vi "replace AO wf param.vi"(0 "Digital Freq (Hz)":dbl, 1 "Digital DC (%)":dbl, 2 "Digital phase":dbl, 3 "Sampling frequency (Hz)":dbl, 4 "Digital time offset (s)":dbl, 5 "index of DO wave":i32, 8 "padding value":dbl) -> ()   [LabVIEW 2015]
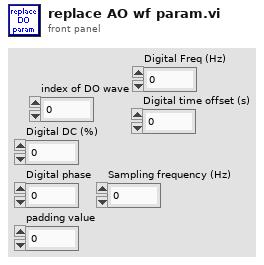
[diagram p1: front panel]
types:
  T1 = cluster{"AO parameters":cluster{"AOtab":dbl, "Repeats":dbl, "Cycles":dbl, "Start amplitude (V)":dbl, "Baseline (V)":dbl, "Step size (V)":dbl, "DC (%)":dbl, "Sampling frequency (Hz)":dbl, "Period (ms)":dbl, "Offset (V)":dbl, "Amplitude (V)":dbl, "Frequency":dbl, "Tri Repeats":dbl, "Cycle length (s)":dbl, "Pulses":dbl, "Matlab wave number":dbl, "Tri phase":dbl, "padding value":dbl}[], "DO parameters":cluster{"Digital DC (%)":dbl, "Digital phase":dbl, "Digital Freq (Hz)":dbl, "Sampling frequency (Hz)":dbl, "Digital time offset (s) ":dbl, "padding value":dbl}[]}
  T2 = cluster{"Digital DC (%)":dbl, "Digital phase":dbl, "Digital Freq (Hz)":dbl, "Sampling frequency (Hz)":dbl, "Digital time offset (s) ":dbl, "padding value":dbl}[]
  T3 = cluster{"Digital DC (%)":dbl, "Digital phase":dbl, "Digital Freq (Hz)":dbl, "Sampling frequency (Hz)":dbl, "Digital time offset (s) ":dbl, "padding value":dbl}
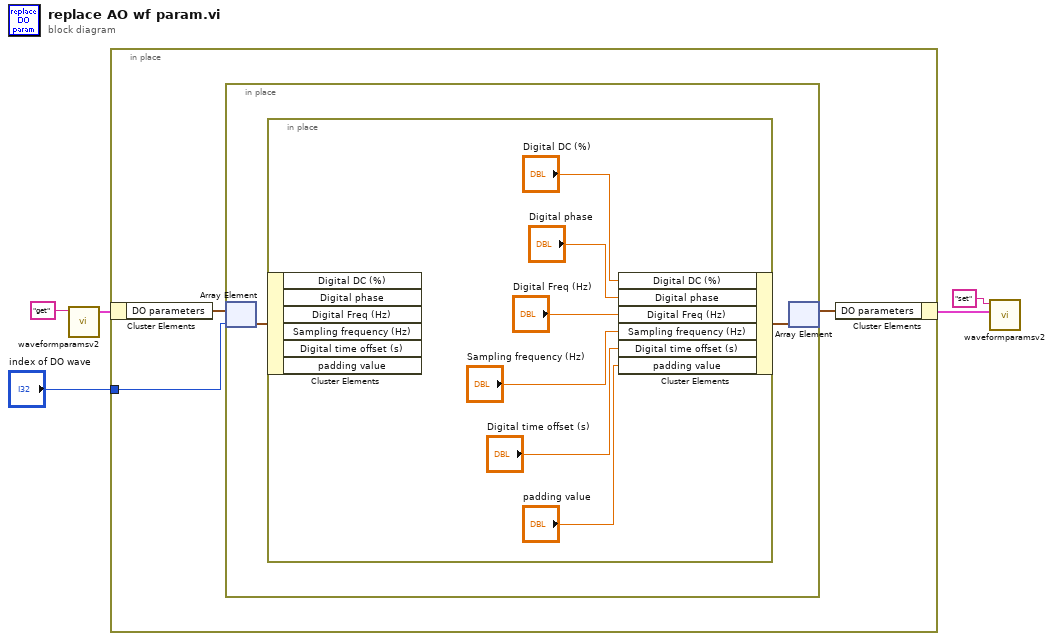
[diagram p0: block diagram]
diagram:
  n1 = call "waveformparamsv2.vi"("command"="get") -> ("Params out"=w3:T1)  [unwired: 4 in, 2 out]
  n2 = in-place {
    in-place-border: "index of DO wave" -> [w6]
    n3 = in-place-cluster #1(w3) -> ("DO parameters"=w8:T2)
    n4 = in-place {
      n5 = in-place-array #2(w8, w6) -> (w10:T3)
      n6 = in-place {
        n7 = in-place-cluster #3(w10) -> ()  [unwired: 6 out]
        n8 = in-place-cluster #3("Digital DC (%)"="Digital DC (%)", "Digital phase"="Digital phase", "Digital Freq (Hz)"="Digital Freq (Hz)", "Sampling frequency (Hz)"="Sampling frequency (Hz)", "Digital time offset (s)"="Digital time offset (s)", "padding value"="padding value") -> (w9:T3)
      }
      n9 = in-place-array #2(w9) -> (w7:T2)  [unwired: 1 out]
    }
    n10 = in-place-cluster #1("DO parameters"=w7) -> (w4:T1)
  }
  n11 = call "waveformparamsv2.vi"("command"="set", "Params in"=w4) -> ()  [unwired: 3 in, 3 out]
